vi "Read Control Label.vi"(8 "error in (no error)":errorcluster, 11 "TreeItemOpenMsg in":refnum<class "TreeItemOpenMsg.lvclass">) -> (0 "error out":errorcluster, 2 "Control Label":string, 3 "TreeItemOpenMsg out":refnum<class "TreeItemOpenMsg.lvclass">)   [LabVIEW 2018, in "MVA Framework.lvlib" / "ActorEvents.lvlib" / "TreeItemOpenMsg.lvclass"]
uses:
  TreeItemOpenMsg.lvclass
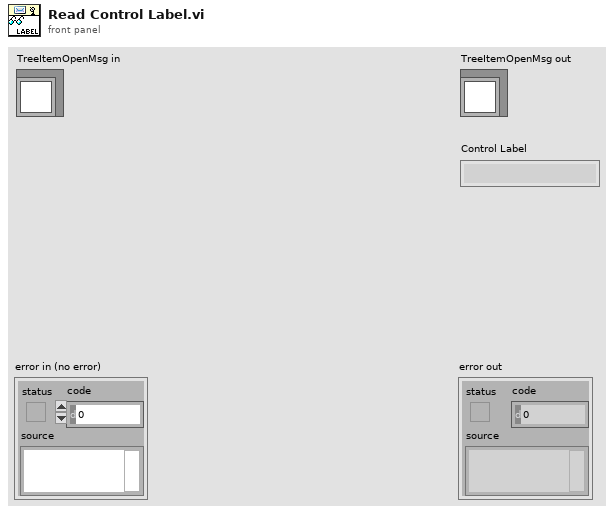
[diagram p1: front panel]
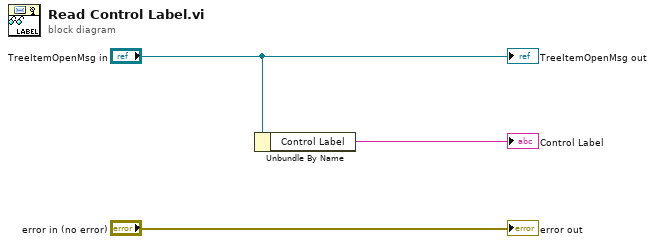
[diagram p0: block diagram]
diagram:
  n1 = Unbundle By Name("TreeItemOpenMsg in") -> ("Control Label"=→"Control Label":string)
  "error out" <- "error in (no error)"
  "TreeItemOpenMsg out" <- "TreeItemOpenMsg in"
